vi "Download Binding.vi"(8 "error in (no error)":errorcluster, 9 "index":i32, 10 "Recipes.Binding":T1(array[cluster]), 11 "Programing Logic in":refnum<class "Programing Logic.lvclass">) -> (0 "error out":errorcluster, 3 "Programing Logic out":refnum<class "Programing Logic.lvclass">)   [LabVIEW 2014, in "Programing Logic.lvclass"]
uses:
  Programing Logic.lvclass
  Programing Logic.lvclass/Programing Logic.ctl
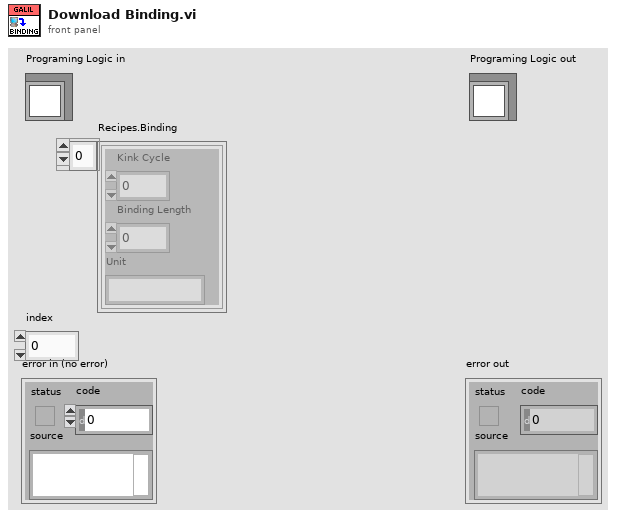
[diagram p1: front panel]
types:
  T1 = cluster{"Kink Cycle":dbl, "Binding Length":dbl, "Unit":string}[]
  T2 = cluster{"Kink Cycle":dbl, "Binding Length":dbl, "Unit":string}
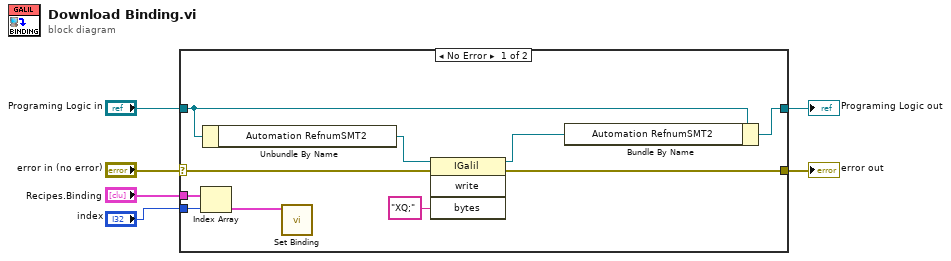
[diagram p0: block diagram]
diagram:
  n1 = case shown="No Error" "error in (no error)" {
    selector: "error in (no error)" -> [w14 w18]
    tunnel: [w13 w18] -> w5
    tunnel: [w10 w17] -> w3
    tunnel: "Programing Logic in" -> [w11 w17]
    tunnel: "index" -> [w16 _]
    tunnel: "Recipes.Binding" -> [w15 _]
    frame No Error {
      n2 = Index Array(array=w15, index=w16) -> (element=w12:T2)
      n3 = Unbundle By Name(w11) -> ("Automation RefnumSMT2"=w9:refnum<k7>)
      n4 = call "Set Binding.vi"("Recipes.Binding"=w12) -> ()  [unwired: 10 in, 1 out]
      n5 = invoke class="IGalil" method="write"(reference=w9, error in=w14, "bytes"="XQ;") -> (reference out=w8:refnum<k7>, error out=w13:errorcluster)  [unwired: 1 in, 2 out]
      n6 = Bundle By Name(cluster=w11, "Automation RefnumSMT2"=w8) -> (w10:refnum<class "Programing Logic.lvclass">)
    }
    frame Error {
    }
  }
  "error out" <- w5
  "Programing Logic out" <- w3
